vi "Compare ShotNumber from MC and Path.vi"(9 "Shot Number":dbl, 10 "DeviceName":string, 11 "Input Path":path) -> (3 "ShotNumberMatch":bool)   [LabVIEW 2020]
uses:
  <userlib>/_OpenG.lib/file/file.llb/Strip Path - Traditional__ogtk.vi
  <vilib>/regexp/Match Regular Expression.xnode
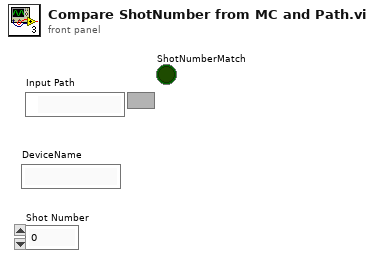
[diagram p1: front panel]
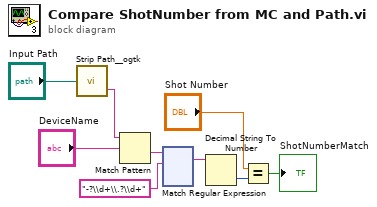
[diagram p0: block diagram]
diagram:
  n1 = call-poly <userlib>:"Strip Path__ogtk.vi"("path"="Input Path") -> ("name"=w8:string)  [unwired: 1 out]
  n2 = Match Pattern(string=w8, regular expression="DeviceName") -> (after substring=w1:string)  [unwired: 1 in, 3 out]
  n3 = xnode "Match Regular Expression"("input string"=w1, "regular expression"="-?\\d+\\.?\\d+") -> ("whole match"=w5:string)  [unwired: 4 in, 4 out]
  n4 = Decimal String To Number(string=w5) -> (number=w4:i32)  [unwired: 2 in, 1 out]
  n5 = Equal?(x="Shot Number", y=w4) -> (x = y?=→"ShotNumberMatch":bool)
